vi "PerfAddRemove.vi"() -> (3 "Add time":dbl format="%.2p")   [LabVIEW 2024, in "POTCircularBuffer.Test.Perf.lvlib"]
uses:
  POTCircularBuffer.Test.Perf.lvlib
  dcabc875-db76-4c53-9c4f-cf505999d426.vi
  6045e48b-d2eb-4048-91f0-a5fde5ba3311.vi
  <vilib>/Analysis/baseanly.llb/Mean (DBL).vi
  10666d2b-b659-4efd-8cbe-8400d97b5c3b.vi
  f3bdf14e-c875-47e4-8bb6-bd7377a45b73.vi
  dcabc875-db76-4c53-9c4f-cf505999d426.vi/861d1239-c00a-4baa-b197-0d315609214a.vi
  internal/Wrap.vi
  10666d2b-b659-4efd-8cbe-8400d97b5c3b.vi/861d1239-c00a-4baa-b197-0d315609214a.vi
  f3bdf14e-c875-47e4-8bb6-bd7377a45b73.vi/83157745-27d4-4525-9754-43251232a38d.vi
  f3bdf14e-c875-47e4-8bb6-bd7377a45b73.vi/b3dbe2ff-c37c-4d84-9589-eb33aa9d1bc4.vi
  f3bdf14e-c875-47e4-8bb6-bd7377a45b73.vi/b3dbe2ff-c37c-4d84-9589-eb33aa9d1bc4.vi/026309cf-e2b3-4d2a-859d-4b9253ede2ce.vi
  f3bdf14e-c875-47e4-8bb6-bd7377a45b73.vi/b3dbe2ff-c37c-4d84-9589-eb33aa9d1bc4.vi/79793457-486d-421b-94da-54962abb47fa.vi
  f3bdf14e-c875-47e4-8bb6-bd7377a45b73.vi/b3dbe2ff-c37c-4d84-9589-eb33aa9d1bc4.vi/0085ecbf-1180-4e84-bda3-723fc83f2dac.vi
  f3bdf14e-c875-47e4-8bb6-bd7377a45b73.vi/b3dbe2ff-c37c-4d84-9589-eb33aa9d1bc4.vi/4f836871-2ac6-4fbb-a4b2-2354c860e67a.vi
  f3bdf14e-c875-47e4-8bb6-bd7377a45b73.vi/b3dbe2ff-c37c-4d84-9589-eb33aa9d1bc4.vi/026309cf-e2b3-4d2a-859d-4b9253ede2ce.vi/83cdeaba-e1ff-493a-b62c-1f93efcfb5e6.vi
  f3bdf14e-c875-47e4-8bb6-bd7377a45b73.vi/b3dbe2ff-c37c-4d84-9589-eb33aa9d1bc4.vi/79793457-486d-421b-94da-54962abb47fa.vi/e824a7ab-ba84-44ad-941c-e55b0f65d782.vi
  f3bdf14e-c875-47e4-8bb6-bd7377a45b73.vi/b3dbe2ff-c37c-4d84-9589-eb33aa9d1bc4.vi/79793457-486d-421b-94da-54962abb47fa.vi/e824a7ab-ba84-44ad-941c-e55b0f65d782.vi/83cdeaba-e1ff-493a-b62c-1f93efcfb5e6.vi
  <vilib>/Analysis/NI_AALBase.lvlib
panel:
  out "remove time":dbl format="%.2p"
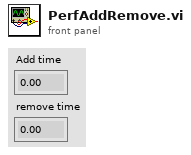
[diagram p1: front panel]
types:
  T1 = cluster{"buffer":u32[], "head":i32, "tail":i32, "size":i32, "capacity":i32, "mask":i32}
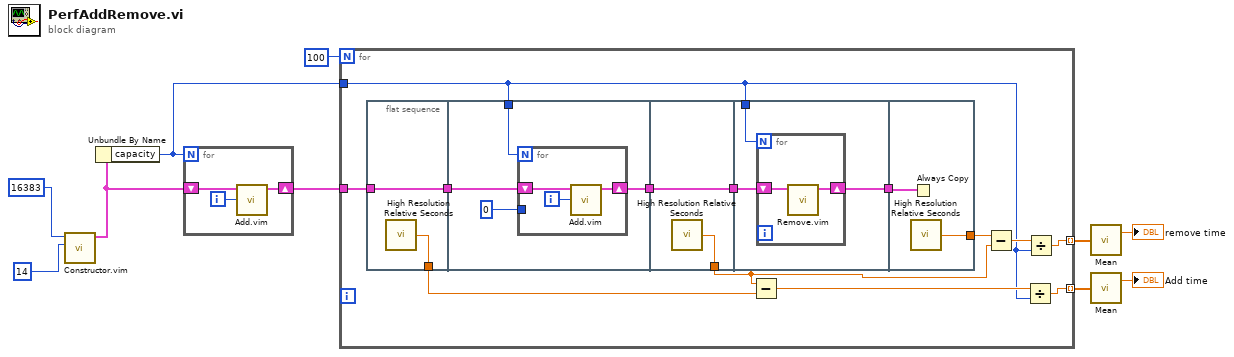
[diagram p0: block diagram]
diagram:
  n1 = call "Constructor.vim"("Capacity 2^n"=u32 14 ("Capacity"), "Placeholder Type"=u32 16383 ("Capacity")) -> ("CircularBuffer out"=w1:T1)  [unwired: 9 in]
  n2 = Unbundle By Name(w1) -> ("capacity"=w4:i32)
  n3 = for {
    N: w4 -> [_]
    shift-right: [w12] -> w5
    shift-left: w1 -> [w13]
    i -> [w11]
    n4 = call "Add.vim"("New Element"=w11, "CircularBuffer in"=w13) -> ("CircularBuffer out"=w12:T1)  [unwired: 9 in]
  }
  n5 = for {
    N: 100 -> [_]
    tunnel: [w18] -> w10 mode=indexing
    tunnel: w5 -> [w25]
    tunnel: [w16] -> w6 mode=indexing
    tunnel: w4 -> [w15]
    n6 = flat-sequence {
      tunnel: w25 -> [w28]
      tunnel: [w28] -> w22
      tunnel: [w27] -> w20
      tunnel: [w31] -> w23
      tunnel: w22 -> [w32]
      tunnel: w15 -> [w29]
      tunnel: [w37] -> w21
      tunnel: [w36] -> w24
      tunnel: w23 -> [w36]
      tunnel: w24 -> [w40]
      tunnel: w15 -> [w39]
      tunnel: [w38] -> w14
      tunnel: [w44] -> w26
      tunnel: w14 -> [w43]
      frame #0 {
        n7 = call <vilib>:"High Resolution Relative Seconds.vi"() -> ("relative seconds"=w27:dbl)
      }
      frame #1 {
        n8 = for {
          N: w29 -> [_]
          shift-right: [w34] -> w31
          shift-left: w32 -> [w35]
          tunnel: u32 0 ("Capacity") -> [_]
          i -> [w33]
          n9 = call "Add.vim"("New Element"=w33, "CircularBuffer in"=w35) -> ("CircularBuffer out"=w34:T1)  [unwired: 9 in]
        }
      }
      frame #2 {
        n10 = call <vilib>:"High Resolution Relative Seconds.vi"() -> ("relative seconds"=w37:dbl)
      }
      frame #3 {
        n11 = for {
          N: w39 -> [_]
          shift-right: [w41] -> w38
          shift-left: w40 -> [w42]
          n12 = call "Remove.vim"("CircularBuffer in"=w42) -> ("CircularBuffer out"=w41:T1)  [unwired: 8 in, 2 out]
        }
      }
      frame #4 {
        n13 = Always Copy(1:w43) -> ()  [unwired: 1 out]
        n14 = call <vilib>:"High Resolution Relative Seconds.vi"() -> ("relative seconds"=w44:dbl)
      }
    }
    n15 = Subtract(x=w21, y=w20) -> (x-y=w17:dbl)
    n16 = Subtract(x=w26, y=w21) -> (x-y=w19:dbl)
    n17 = Divide(x=w17, y=w15) -> (x/y=w16:dbl)
    n18 = Divide(x=w19, y=w15) -> (x/y=w18:dbl)
  }
  n19 = call-poly <vilib>:"Mean.vi"("X"=w10) -> ("mean"=→"remove time":dbl)  [unwired: 1 out]
  n20 = call-poly <vilib>:"Mean.vi"("X"=w6) -> ("mean"=→"Add time":dbl)  [unwired: 1 out]
